vi "CRYCheck TS After TS Read.vi"() -> ()   [LabVIEW 2013]
uses:
  CRYCurveLibrary/Global/CRYCurve Library Global.vi
  CRYProject Editor Global.vi
panel:
  in  "Hardware In":string
  out "Proper VI No":i32
  # "Check TS Component."
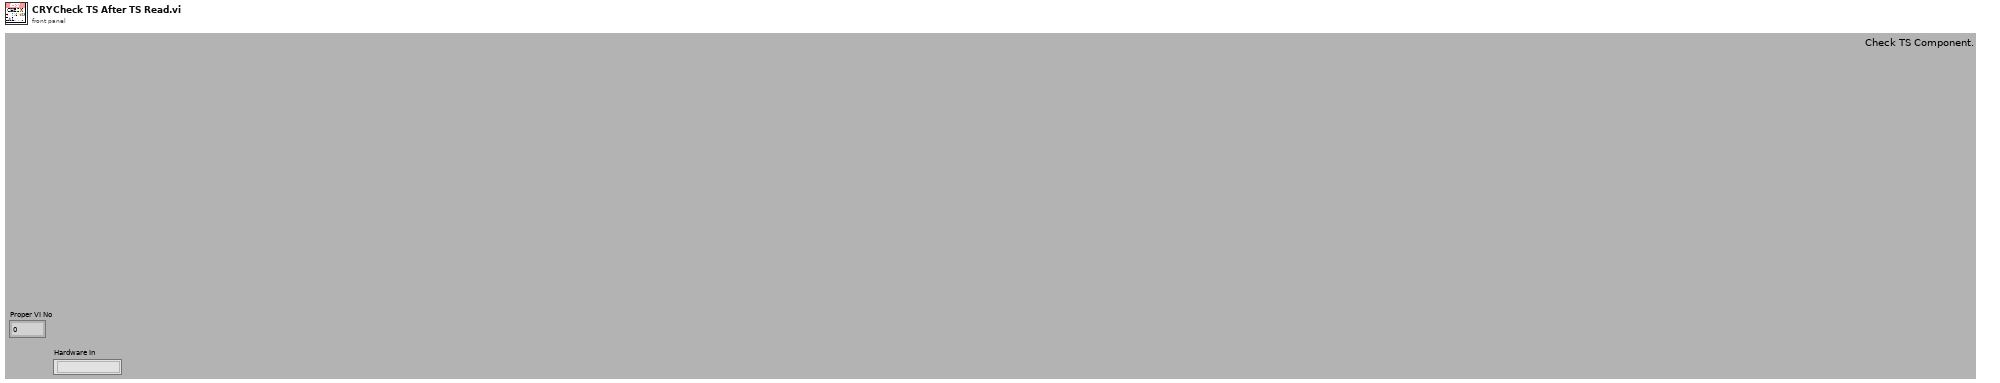
[diagram p1: front panel]
types:
  T1 = typedef "CRYStep.ctl" = cluster{"No.VI":i32, "Category":string, "StepName":string, "Seq setup flattened":string, "Comment":string, "Steps config.":bool[], "Jump config":i32[], "Start":dbl, "Increment":dbl, "Name":string, "Unit":string, "Y data":u16, "Y prefix":string, "Y dB ref":dbl, "Y unit":string, "Repeat State Array":cluster{"Start":dbl, "Increment":dbl, "Count":i32, "Num":i32}[]}
  T2 = typedef "CRYCalibration All Cluster.ctl" = cluster{"Calibration 2D":T3[], "Help":string, "Tab Value":i32, "Input Signal Type":string, "Output Signal Type":string}
  T3 = typedef "CRYCalibration 2DCluster.ctl" = cluster{"Calibration":T4, "Corr Curve":T5, "EQ Curve":T5, "Sens Curve":T5}
  T4 = typedef "CRYCalibration Cluster.ctl" = cluster{"Calibration Step Name":string, "Device":string, "Correction Curve Name":string, "Equalization Curve Name":string, "Sensitivity Curve Name":string, "Corr Folder and File":string, "EQ Folder and File":string, "Sens Folder and File":string, "Corr Step size":u16, "EQ Step size":u16, "Input":bool, "Last Cal Date (sec)":timestamp, "Cha Name":string, "Corr Curve Found":bool, "EQ Curve Found":bool, "Sens Curve Found":bool, "Signal Type":string, "Calibrated Device":string, "Hz":u32}
  T5 = typedef "CRYData Cluster.ctl" = cluster{"Name":string, "Curve":cluster{"x":dbl, "y":dbl, "z":dbl}[], "X data":u16, "Y data":u16, "Z data":u16, "X axis":u16, "Y axis":u16, "Z axis":u16, "X unit":string, "Y unit":string, "Z unit":string, "X dB ref":dbl, "Y dB ref":dbl, "Z dB ref":dbl, "single val":bool, "protected":bool, "display X":bool, "display Y":bool, "display Z":bool, "Test Info":string, "Step No.":i32, "Plot Settings":cluster{"Color":u32, "Interpolation":u8, "Point Style":u8, "Line Style":u8, "Point Color":u32, "Line Width":u8, "Bar Plot Style":u8, "Fill To":i16}, "AutoProtect":bool}
  T6 = typedef "CRYHardware.ctl" = cluster{"Name":string, "Analog I/O":u16, "Digital I/O":u16, "Channels":u8, "Dig Dev ID":u8, "N ports":u8, "Interface":u32, "Dig I/O Ports":cluster{"port #":i16, "width":i16, "direction":i32}[], "Interf settings":cluster{"Type":u16, "COM Port":u8, "Baud rate":u32, "Data bits":u32, "Parity":u16, "Stop bits":u16, "Flow control":u16, "Dev ID IEEE":u8}[], "N interfs":i32, "udev SNs":i16[], "udev enable":bool, "Channel Array":T7[], "Cal sequence":string, "SelectedIn":u16, "SelectedOut":u16, "SelectedTab":u16, "State":bool, "Help":string, "Advanced":bool, "In Audio Driver":u16, "Out Audio Driver":u16}
  T7 = typedef "CRYHardware Channel Info.ctl" = cluster{"ID":i32, "Name":string, "Digital":bool, "Input":bool, "Device Name":string, "Hardware Ch ID":u8, "Vmax (V)":dbl, "Latency (samples)":dbl, "Sampling Rate (Hz)":u32, "Bit Depth":u32, "Anti-aliasing Factor (%fs)":sgl, "DAQmx Channel":tag, "term config":i32, "Coupling":i32, "IEPE en":bool, "ASIOChannel Name":string, "Audio Driver":u16, "ASIOChannel Index":u8}
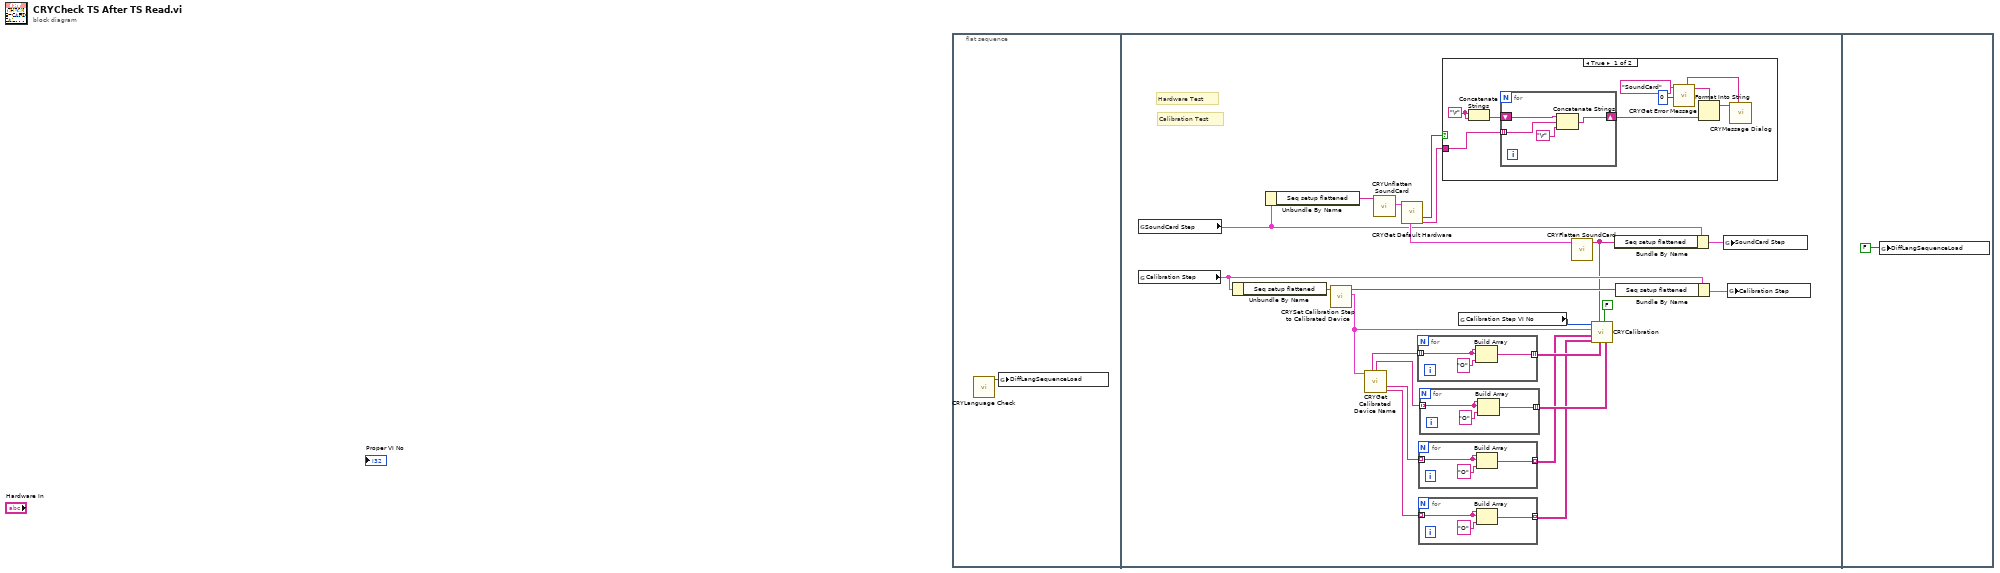
[diagram p0: block diagram]
diagram:
  n1 = flat-sequence {
    frame #0 {
      n2 = call "CRYLanguage Check.vi"() -> ("DiffLanguage"=w1:bool)  [unwired: 10 in, 1 out]
      n3 = global write "CRYCurve Library Global.vi" "DiffLangSequenceLoad"(w1) -> ()
    }
    frame #1 {
      # "Calibration Test"
      # "Hardware Test"
      n4 = global read "CRYProject Editor Global.vi" "SoundCard Step"() -> (w18:T1)
      n5 = global read "CRYProject Editor Global.vi" "Calibration Step"() -> (w17:T1)
      n6 = Unbundle By Name(w17) -> ("Seq setup flattened"=w19:string)
      n7 = Unbundle By Name(w18) -> ("Seq setup flattened"=w23:string)
      n8 = call "CRYSet Calibration Step to Calibrated Device.vi"("Calibration setup In"=w19) -> ("output Calibration"=w15:T2, "Calibration flattened out"=w16:string)  [unwired: 9 in]
      n9 = call "CRYGet Calibrated Device Name.vi"("Calibration"=w15) -> ("I_Signal Type Out"=w12:string[], "O_Signal Type Out"=w11:string[], "I_Calibrated Device Out"=w8:string[], "O_Calibrated Device Out"=w7:string[])  [unwired: 7 in, 4 out]
      n10 = call "CRYUnflatten SoundCard.vi"("Flatten SoundCard"=w23) -> ("SoundCard"=w24:T6)  [unwired: 10 out]
      n11 = call "CRYGet Default Hardware.vi"("Hardware Cluster In"=w24) -> ("Hardware Cluster Out"=w20:T6, "Error"=w22:bool, "No Device Name"=w21:string[])  [unwired: 16 out]
      n12 = for {
        tunnel: w12 -> [w36] mode=indexing
        tunnel: [w34] -> w10 mode=indexing
        n13 = Build Array(w36, w36, "O" ("element")) -> (w34:string[])
      }
      n14 = for {
        tunnel: w8 -> [w30] mode=indexing
        tunnel: [w28] -> w6 mode=indexing
        n15 = Build Array(w30, w30, "O" ("element")) -> (w28:string[])
      }
      n16 = for {
        tunnel: w7 -> [w27] mode=indexing
        tunnel: [w25] -> w5 mode=indexing
        n17 = Build Array(w27, w27, "O" ("element")) -> (w25:string[])
      }
      n18 = for {
        tunnel: w11 -> [w33] mode=indexing
        tunnel: [w31] -> w9 mode=indexing
        n19 = Build Array(w33, w33, "O" ("element")) -> (w31:string[])
      }
      n20 = case shown="True" w22 {
        tunnel: w21 -> [w40 _]
        frame True {
          w38 = "\r"
          n21 = Concatenate Strings(w38, w38) -> (w37:string)
          n22 = for {
            tunnel: w40 -> [w48] mode=indexing
            shift-right: [w46] -> w39
            shift-left: w37 -> [w49]
            n23 = Concatenate Strings(w49, w48, "\r") -> (w46:string)
          }
          n24 = call "CRYGet Error Message.vi"("Error No"=0 ("No"), "Kind"="SoundCard") -> ("Message"=w43:string, "Window Title"=w42:string)  [unwired: 4 in, 4 out]
          n25 = Format Into String(format string=w43, w39) -> (resulting string=w41:string)  [unwired: 2 in, 1 out]
          n26 = call "CRYMessage Dialog.vi"("Window Title"=w42, "Message Content"=w41) -> ()  [unwired: 8 in, 2 out]
        }
        frame False {
        }
      }
      n27 = global read "CRYProject Editor Global.vi" "Calibration Step VI No"() -> (w3:i32)
      n28 = call "CRYFlatten SoundCard.vi"("SoundCard"=w20) -> ("SoundCard flattened"=w14:string)  [unwired: 10 out]
      n29 = call "CRYCalibration.vi"("O_Signal Type Old In"=w9, "Apply?"=FALSE, "I_Signal Type Old In"=w10, "Hardware In"=w14, "O_Calibrated Device Name Old In"=w5, "I_Calibrated Device Name Old In"=w6, "Calibration"=w15, "Proper VI No In"=w3) -> ()  [unwired: 4 out]
      n30 = Bundle By Name(cluster=w18, "Seq setup flattened"=w14) -> (w2:T1)
      n31 = Bundle By Name(cluster=w17, "Seq setup flattened"=w16) -> (w4:T1)
      n32 = global write "CRYProject Editor Global.vi" "SoundCard Step"(w2) -> ()
      n33 = global write "CRYProject Editor Global.vi" "Calibration Step"(w4) -> ()
    }
    frame #2 {
      n34 = global write "CRYCurve Library Global.vi" "DiffLangSequenceLoad"(FALSE ("SequenceLoad")) -> ()
    }
  }
